vi "scott -- strain -- 150220 -- Strain SC Main -- V0.vi"(8 "error in":errorcluster, 9 "temperature":dbl=114.59, 10 "sweep folder name":path=path "D:/Technique/Strain/URu2Si2-xPx/x=0.01/141113 URu2Si2 0p01 eyy ryy.dat", 11 "strain sweep control":T1={"just in case"=TRUE, "Piezo Amplifier settings"={"Gain "=69.44, "offset (V)"=69.44}, "voltage-parameters-IN"={"phase "=2.88, "amplitude (V)"=-0.7854, "offset (V)"=0.28, "time delay (sec)"=0.5, "period (sec)"=50.0, "shape"=enum."triangle"}, "Lockin Settings"=[{"Offset"=FALSE, "GPIB Address"=6}, {"Offset"=TRUE, "GPIB Address"=7}], "VISA address Agilent  IN"="", "number of iterations"=1.0, "Piezo sweep settings"={"max Piezo voltage (V) "=69.44, "min Piezo voltage (V)"=69.44, "delay (sec)"=69.44, "period (sec)"=69.44, "shape"=enum."triangle"}}) -> (0 "error out":errorcluster)   [LabVIEW 2014]
uses:
  Scott -- strain -- strain sweep control.ctl
  FSU/ScottRiggs/Piezo2/voltage-wave-generator-parameters.ctl
  FSU/ScottRiggs/Piezo/votage-control.ctl
panel:
  in  "Tab Control":enum32{"Elasto-resistivity", "Graphs 1-2"}(tab)
  out "total number of points":dbl=114.59
  out "voltage out (V)":dbl=114.59
  out "Agilent OK!":bool
  out "Lockin 1 Graph":cluster{"X Data":dbl[], "Y Data":dbl[]}[](graph)=[{"X Data"=array[300 elements], "Y Data"=array[300 elements]}, {"X Data"=array[300 elements], "Y Data"=[0.34598, 0.34601, 0.34601, 0.34598, 0.34598, 0.34598, 0.34598, 0.34598, 0.34598, 0.34598, 0.34598, 0.34598, 0.34598, 0.345949, 0.34598, 0.34598, 0.34598, 0.34598, 0.34598, 0.34598, 0.34598, 0.34598, 0.34598, 0.34598, 0.34598, 0.34598, 0.34598, 0.34598, 0.34598, 0.34598, 0.34598, 0.34598, 0.34598, 0.34601, 0.34601, 0.34601, 0.34601, 0.34601, 0.34601, 0.34601, 0.34601, 0.34601, 0.34601, 0.34601, 0.34601, 0.34601, 0.34601, 0.346041, 0.346041, 0.346041, 0.346041, 0.346041, 0.346041, 0.346041, 0.346041, 0.346071, 0.346071, 0.346071, 0.346071, 0.346071, 0.346071, 0.346071, 0.346071, 0.346071, 0.346071, 0.346071, 0.346071, 0.346071, 0.346071, 0.346071, 0.346071, 0.346071, 0.346071, 0.346071, 0.346041, 0.346071, 0.346071, 0.346071, 0.346041, 0.346041, 0.346041, 0.346041, 0.346041, 0.34601, 0.346041, 0.346041, 0.34601, 0.34601, 0.34601, 0.34601, 0.34601, 0.34601, 0.34601, 0.34601, 0.34601, 0.34601, 0.34601, 0.34601, 0.34601, 0.34598, 0.34598, 0.34598, 0.34601, 0.34598, 0.34598, 0.34598, 0.34598, 0.34598, 0.34598, 0.34598, 0.34598, 0.34598, 0.34598, 0.34598, 0.34598, 0.34598, 0.34598, 0.34598, 0.34598, 0.34598, 0.34598, 0.34598, 0.34598, 0.34598, 0.34598, 0.34598, 0.34598, 0.34598, 0.34598, 0.34598, 0.34598, 0.34598, 0.34598, 0.34601, 0.34601, 0.34601, 0.34601, 0.34601, 0.34601, 0.34601, 0.34601, 0.34601, 0.34601, 0.34601, 0.34601, 0.34601, 0.346041, 0.346041, 0.34601, 0.34601, 0.346041, 0.346041, 0.346041, 0.346041, 0.346041, 0.346071, 0.346071, 0.346041, 0.346071, 0.346071, 0.346071, 0.346071, 0.346071, 0.346071, 0.346071, 0.346071, 0.346071, 0.346071, 0.346071, 0.346071, 0.346071, 0.346071, 0.346041, 0.346041, 0.346071, 0.346041, 0.346041, 0.346041, 0.346041, 0.346041, 0.346041, 0.34601, 0.346041, 0.346041, 0.34601, 0.34601, 0.34601, 0.34601, 0.34601, 0.34601, 0.34601, 0.34601, 0.34601, 0.34601, 0.34601, 0.34601, 0.34601, 0.34601, 0.34598, 0.34598, 0.34598, 0.34598, 0.34598, 0.34598, 0.34598, 0.34598, 0.34598, 0.34598, 0.34598, 0.34598, 0.34598, 0.34598, 0.34598, 0.34598, 0.34598, 0.345949, 0.34598, 0.34598, 0.34598, 0.34598, 0.34598, 0.34598, 0.34598, 0.34598, 0.34598, 0.34598, 0.34598, 0.34598, 0.34598, 0.34598, 0.34601, 0.34601, 0.34601, 0.34601, 0.34601, 0.34601, 0.34601, 0.34601, 0.34601, 0.34601, 0.34601, 0.34601, 0.34601, 0.34601, 0.34601, 0.34601, 0.34601, 0.346041, 0.346041, 0.346041, 0.346041, 0.346041, 0.346071, 0.346071, 0.346041, 0.346041, 0.346071, 0.346071, 0.346071, 0.346071, 0.346071, 0.346071, 0.346071, 0.346071, 0.346071, 0.346071, 0.346071, 0.346071, 0.346071, 0.346071, 0.346071, 0.346071, 0.346071, 0.346071, 0.346071, 0.346071, 0.346071, 0.346071, 0.346071, 0.346041, 0.346041, 0.346041, 0.346041, 0.346041, 0.34601, 0.346041, 0.346041, 0.34601, 0.34601, 0.34601, 0.34601, 0.34601, 0.34601, 0.34601, 0.34601, 0.34601, 0.34601, 0.34601, 0.34601, 0.34601]}, {"X Data"=array[300 elements], "Y Data"=array[300 elements]}, {"X Data"=array[300 elements], "Y Data"=[0.018135, 0.018139, 0.018133, 0.018133, 0.018137, 0.018135, 0.018133, 0.018133, 0.018131, 0.018129, 0.018129, 0.018127, 0.018131, 0.018131, 0.018127, 0.018127, 0.018127, 0.018125, 0.018127, 0.018127, 0.018123, 0.018129, 0.018131, 0.018127, 0.018135, 0.018139, 0.018139, 0.01814, 0.01814, 0.018137, 0.018131, 0.018131, 0.018127, 0.018137, 0.01814, 0.018139, 0.018135, 0.018133, 0.018139, 0.018135, 0.018139, 0.018144, 0.018142, 0.01814, 0.018144, 0.01815, 0.018144, 0.018146, 0.01814, 0.018139, 0.018135, 0.018129, 0.018129, 0.018135, 0.018142, 0.01814, 0.01814, 0.018142, 0.018146, 0.018144, 0.018144, 0.01815, 0.018144, 0.01814, 0.01814, 0.018137, 0.018137, 0.018137, 0.01814, 0.01814, 0.018137, 0.018131, 0.018131, 0.018137, 0.018137, 0.018144, 0.01814, 0.018131, 0.018131, 0.018129, 0.018131, 0.018139, 0.018148, 0.018144, 0.018139, 0.018133, 0.018131, 0.018133, 0.018127, 0.018129, 0.018119, 0.018123, 0.018125, 0.018127, 0.018133, 0.018133, 0.018131, 0.018129, 0.018131, 0.018133, 0.018129, 0.018129, 0.018131, 0.018133, 0.018127, 0.018123, 0.018121, 0.018125, 0.018127, 0.018131, 0.018129, 0.018127, 0.018127, 0.018127, 0.018129, 0.018123, 0.018127, 0.018125, 0.018116, 0.018116, 0.018127, 0.018127, 0.018123, 0.018121, 0.018125, 0.018127, 0.018127, 0.018127, 0.018135, 0.018135, 0.018129, 0.018131, 0.018125, 0.018118, 0.018121, 0.018135, 0.018139, 0.01814, 0.018146, 0.018142, 0.01814, 0.018137, 0.018127, 0.018127, 0.018135, 0.01814, 0.01814, 0.018137, 0.018127, 0.018133, 0.018137, 0.018142, 0.018142, 0.01814, 0.01814, 0.01814, 0.018142, 0.01814, 0.018135, 0.01814, 0.01814, 0.018135, 0.018139, 0.018139, 0.01814, 0.01814, 0.018146, 0.018146, 0.01814, 0.018144, 0.018146, 0.018144, 0.018139, 0.018139, 0.018135, 0.018137, 0.01814, 0.01814, 0.018139, 0.018131, 0.018139, 0.018139, 0.018133, 0.018135, 0.018129, 0.018131, 0.018137, 0.018133, 0.018135, 0.018139, 0.018139, 0.018137, 0.018133, 0.018129, 0.018129, 0.018125, 0.018129, 0.018135, 0.018133, 0.018135, 0.018125, 0.018127, 0.018123, 0.018125, 0.018127, 0.018127, 0.018125, 0.018125, 0.018125, 0.018125, 0.018127, 0.018127, 0.018133, 0.018129, 0.018129, 0.018127, 0.018123, 0.018131, 0.018129, 0.018129, 0.018133, 0.018131, 0.018137, 0.018137, 0.018135, 0.018135, 0.018129, 0.018133, 0.018137, 0.018135, 0.018131, 0.018129, 0.018131, 0.018135, 0.018139, 0.01814, 0.018139, 0.018139, 0.018129, 0.018131, 0.01814, 0.018127, 0.018131, 0.018133, 0.018129, 0.018131, 0.018137, 0.018131, 0.018135, 0.01814, 0.018139, 0.018135, 0.018135, 0.018133, 0.018137, 0.018139, 0.018137, 0.018133, 0.01814, 0.01814, 0.018133, 0.018133, 0.018133, 0.01814, 0.018146, 0.018148, 0.018142, 0.01814, 0.01814, 0.018135, 0.018131, 0.01814, 0.01814, 0.01814, 0.01814, 0.01814, 0.018135, 0.018133, 0.018139, 0.018133, 0.018129, 0.018135, 0.018133, 0.018135, 0.018135, 0.018135, 0.018137, 0.018135, 0.018135, 0.018135, 0.018131, 0.018131, 0.018125, 0.018125, 0.018129, 0.018129, 0.018127, 0.018125, 0.018121, 0.018118]}] caption="XY Graph"
  in  "plots control":cluster{"data string in":string, bool, bool}[](array[cluster])
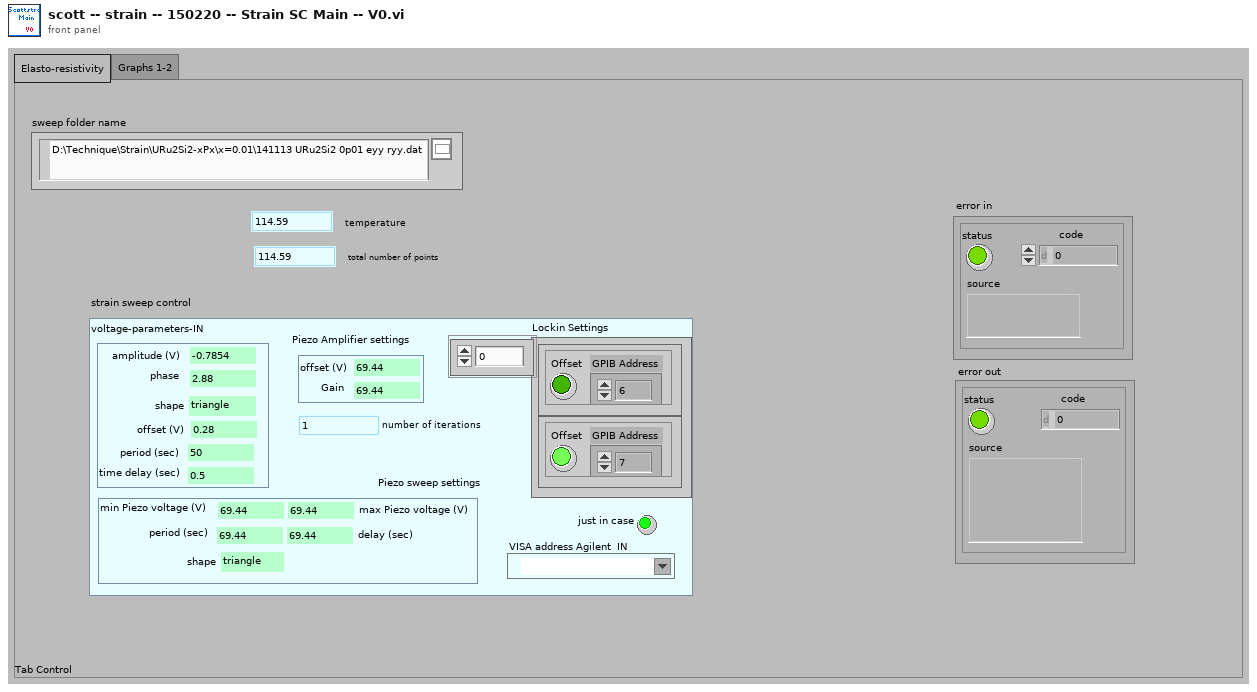
[diagram p1: front panel]
types:
  T1 = typedef "Scott -- strain -- strain sweep control.ctl" = cluster{"just in case":bool, "Piezo Amplifier settings":cluster{"Gain ":dbl, "offset (V)":dbl}, "voltage-parameters-IN":T2, "Lockin Settings":cluster{"Offset":bool, "GPIB Address":i16}[], "VISA address Agilent  IN":refnum<visa-resource-name>, "number of iterations":dbl, "Piezo sweep settings":cluster{"max Piezo voltage (V) ":dbl, "min Piezo voltage (V)":dbl, "delay (sec)":dbl, "period (sec)":dbl, "shape":enum16{"triangle", "sine", "none"}}}
  T2 = typedef "voltage-wave-generator-parameters.ctl" = cluster{"phase ":dbl, "amplitude (V)":dbl, "offset (V)":dbl, "time delay (sec)":dbl, "period (sec)":dbl, "shape":enum16{"triangle", "sine", "none"}}
  T3 = typedef "votage-control.ctl" = enum16{"reset", "next", "use index"}
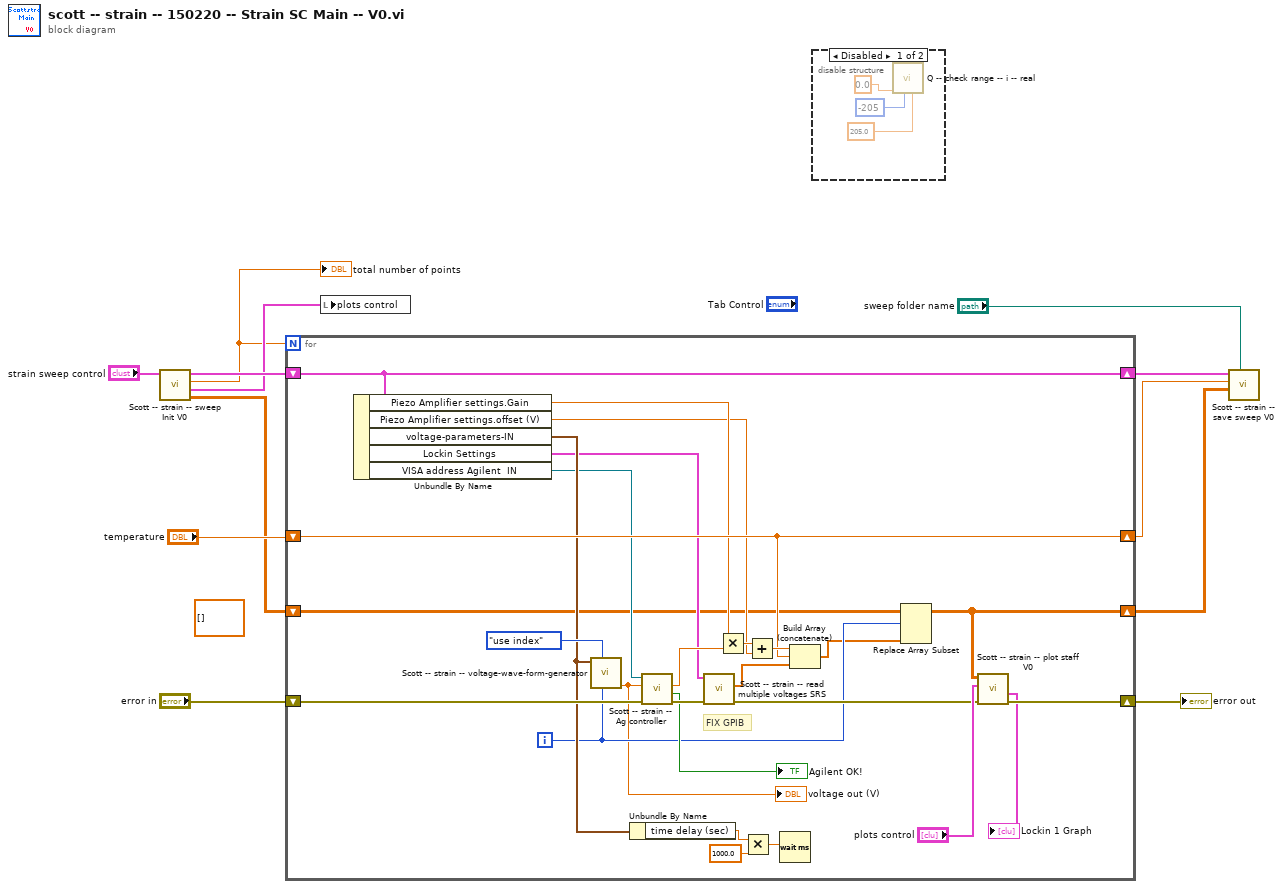
[diagram p0: block diagram]
diagram:
  (unwired) dbl[][] []
  n1 = call "Scott -- strain -- sweep Init V0.vi"("strain sweep control"="strain sweep control") -> ("data array"=w2:dbl[][], "plots control OUT"=w3:cluster{"data string in":string, bool, bool}[], "total number of points"=w1:dbl, "strain sweep control OUT"=w4:T1)  [unwired: 7 in]
  "total number of points" <- w1
  n2 = for {
    N: w1 -> [_]
    shift-right: [w14] -> w8
    shift-left: w2 -> [w17]
    shift-right: [w31] -> w7
    shift-left: "temperature" -> [w31]
    shift-right: [w28] -> w11
    shift-left: "error in" -> [w27]
    shift-right: [w24] -> w6
    shift-left: w4 -> [w24]
    i -> [w16]
    # "FIX GPIB"
    n3 = Unbundle By Name(w24) -> ("Piezo Amplifier settings.Gain"=w23:dbl, "Piezo Amplifier settings.offset (V)"=w22:dbl, "voltage-parameters-IN"=w21:T2, "Lockin Settings"=w19:cluster{"Offset":bool, "GPIB Address":i16}[], "VISA address Agilent  IN"=w20:refnum<visa-resource-name>)
    n4 = call "Scott -- strain -- voltage-wave-form-generator.vi"("index"=w16, "voltage-wave-control"=votage-control."use index", "voltage-parameters-IN"=w21) -> ("voltage out (V)"=w13:dbl)  [unwired: 6 in, 2 out]
    "voltage out (V)" <- w13
    n5 = Unbundle By Name(w21) -> ("time delay (sec)"=w39:dbl)
    n6 = call "Scott -- strain -- Ag controller.vi"("error in (no error)"=w27, "voltage IN"=w13, "VISA resource name IN"=w20) -> ("error out"=w33:errorcluster, "No Errror!"=→"Agilent OK!":bool, "voltage OUT"=w34:dbl)  [unwired: 5 in, 1 out]
    n7 = call "Scott -- strain -- read multiple voltages SRS.vi"("error IN"=w33, "Lockin Settings IN"=w19) -> ("error OUT"=w29:errorcluster, "voltages"=w32:dbl[])  [unwired: 8 in]
    n8 = Multiply(x=w23, y=w34) -> (x*y=w38:dbl)
    n9 = Multiply(x=w39, y=1000.0) -> (x*y=w36:dbl)
    n10 = Add(x=w38, y=w22) -> (x+y=w37:dbl)
    n11 = Wait (ms)(milliseconds to wait=w36) -> ()  [unwired: 1 out]
    n12 = Build Array (concatenate)(w37, w31, w32) -> (w15:dbl[])
    n13 = Replace Array Subset(array=w17, new element=w15, index (row)=w16) -> (w14:dbl[][])  [unwired: 1 in]
    n14 = call "Scott -- strain -- plot staff V0.vi"("error IN"=w29, "plots control"="plots control", "data"=w14) -> ("error out"=w28:errorcluster, "Lockin 1 Graph"=→"Lockin 1 Graph":cluster{"X Data":dbl[], "Y Data":dbl[]}[])  [unwired: 7 in]
  }
  "error out" <- w11
  n15 = local write "plots control"(w3) -> ()
  n16 = disable-structure shown="Disabled" {
    frame Disabled {
      n17 = call "Q -- check range -- i -- real.vi"("upper"=205.0, "lower"=-205, "default"=0.0) -> ("number in range"=w40:dbl, "number"=w42:dbl)  [unwired: 5 in, 2 out]
    }
    frame Enabled {
    }
  }
  n18 = call "Scott -- strain -- save sweep V0.vi"("sweep folder name"="sweep folder name", "data"=w8, "temperature"=w7, "strain sweep control"=w6) -> ()  [unwired: 8 in]
